vi "substring to double precision long.vi"(9 "String Input":string, 10 "Length":i32, 11 "Offset":i32) -> (3 "Numeric":dbl)   [LabVIEW 2026]
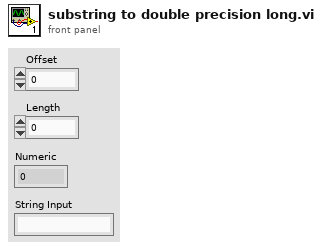
[diagram p1: front panel]
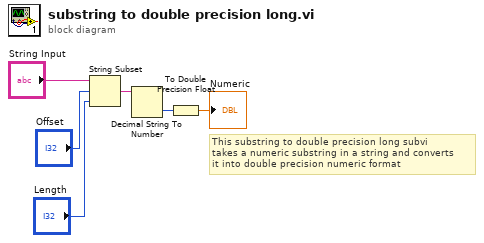
[diagram p0: block diagram]
diagram:
  # "This substring to double precision long subvi\ntakes a numeric substring in a string and converts\nit into double precision numeric format"
  n1 = String Subset(string="String Input", offset (0)="Offset", length (rest)="Length") -> (substring=w5:string)
  n2 = Decimal String To Number(string=w5) -> (number=w4:i32)  [unwired: 2 in, 1 out]
  n3 = To Double Precision Float(number=w4) -> (double precision float=→"Numeric":dbl)
